vi "Soft Start.vi"(3 "Y-axis Joystick":dbl(slide) scale=-1.0..1.0, 4 "Y-Slew Rate":dbl=0.05, 5 "X-Slew Rate":dbl=0.05, 6 "X- axis Joystick":dbl(slide) scale=-1.0..1.0) -> (0 "Y-axis drive":dbl, 2 "X-axis drive":dbl)   [LabVIEW 2014]
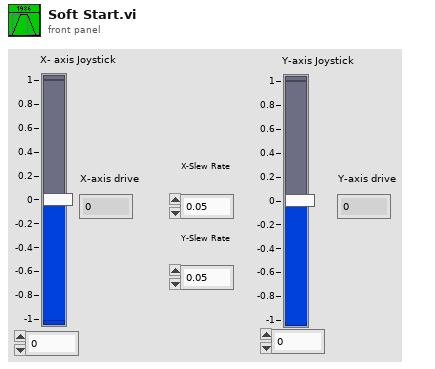
[diagram p1: front panel]
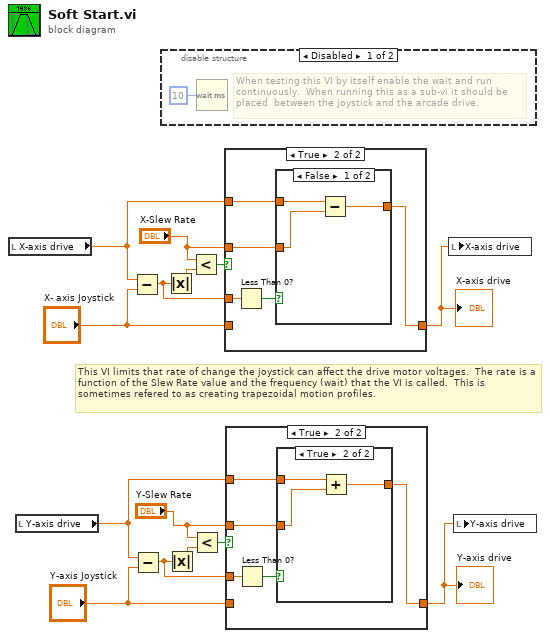
[diagram p0: block diagram]
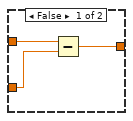
[diagram p4: hidden frame]
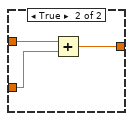
[diagram p6: hidden frame]
diagram:
  # "This VI limits that rate of change the joystick can affect the drive motor voltages.  The rate is a function of the Slew Rate value and the frequency (wait) that the VI is called.  This is sometimes refered to as creating trapezoidal motion profiles."
  n1 = local read "X-axis drive"() -> (w9:dbl)
  n2 = local read "Y-axis drive"() -> (w3:dbl)
  n3 = Subtract(x=w9, y="X- axis Joystick") -> (x-y=w11:dbl)
  n4 = Subtract(x=w3, y="Y-axis Joystick") -> (x-y=w5:dbl)
  n5 = disable-structure shown="Disabled" {
    frame Disabled {
      # "When testing this VI by itself enable the wait and run continuously.  When running this as a sub-vi it should be placed  between the joystick and the arcade drive."
      n6 = Wait (ms)(milliseconds to wait=u32 10) -> ()  [unwired: 1 out]
    }
    frame Enabled {
    }
  }
  n7 = Absolute Value(x=w11) -> (abs(x)=w14:dbl)
  n8 = Absolute Value(x=w5) -> (abs(x)=w8:dbl)
  n9 = Less?(x="X-Slew Rate", y=w14) -> (x < y?=w13:bool)
  n10 = Less?(x="Y-Slew Rate", y=w8) -> (x < y?=w7:bool)
  n11 = case shown="True" w13 {
    tunnel: [w16 w17] -> w10
    tunnel: "X- axis Joystick" -> [w16 _]
    tunnel: w11 -> [_ w21]
    tunnel: w9 -> [_ w19]
    tunnel: "X-Slew Rate" -> [_ w18]
    frame False {
    }
    frame True {
      n12 = Less Than 0?(x=w21) -> (x < 0?=w20:bool)
      n13 = case shown="False" w20 {
        tunnel: w19 -> [w24 w27]
        tunnel: w18 -> [w22 w25]
        tunnel: [w23 w26] -> w17
        frame False {
          n14 = Subtract(x=w24, y=w22) -> (x-y=w23:dbl)
        }
        frame True {
          n15 = Add(x=w27, y=w25) -> (x+y=w26:dbl)
        }
      }
    }
  }
  "X-axis drive" <- w10
  n16 = case shown="True" w7 {
    tunnel: [w28 w29] -> w4
    tunnel: "Y-axis Joystick" -> [w28 _]
    tunnel: w5 -> [_ w33]
    tunnel: w3 -> [_ w31]
    tunnel: "Y-Slew Rate" -> [_ w30]
    frame False {
    }
    frame True {
      n17 = Less Than 0?(x=w33) -> (x < 0?=w32:bool)
      n18 = case shown="True" w32 {
        tunnel: w31 -> [w36 w39]
        tunnel: w30 -> [w34 w37]
        tunnel: [w35 w38] -> w29
        frame False {
          n19 = Subtract(x=w36, y=w34) -> (x-y=w35:dbl)
        }
        frame True {
          n20 = Add(x=w39, y=w37) -> (x+y=w38:dbl)
        }
      }
    }
  }
  "Y-axis drive" <- w4
  n21 = local write "X-axis drive"(w10) -> ()
  n22 = local write "Y-axis drive"(w4) -> ()
